vi "Run Tests.vi"(8 "error in (no error)":errorcluster, 10 "Test Cases":refnum<class "Test Case.lvclass">[](array[class]), 11 "LVUnit Test Executor in":refnum<class "LVUnit Test Executor.lvclass">) -> (0 "error out":errorcluster, 2 "Test Results":refnum<class "Test Result.lvclass">[](array[class]), 3 "LVUnit Test Executor out":refnum<class "LVUnit Test Executor.lvclass">)   [LabVIEW 2017, in "LVUnit Test Executor.lvclass"]
doc: "Runs the specified tests."
uses:
  LVUnit Test Executor.lvclass
  Test Case/Test Case.lvclass
  Test Result/Test Result.lvclass
  Test Outcome.ctl
  Test Result/Test Result.lvclass/Test Result.ctl
  Test Result/Set Outcome.vi
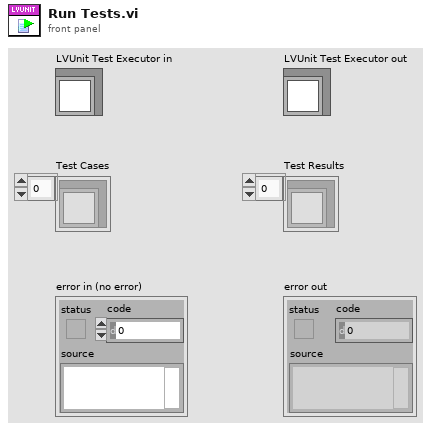
[diagram p1: front panel]
types:
  T1 = typedef "Test Outcome.ctl" = enum16{"None", "Passed", "Failed"}
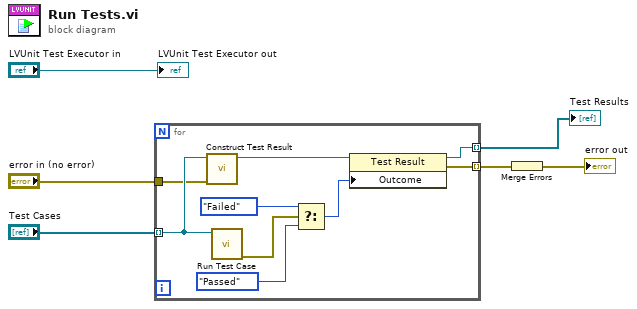
[diagram p0: block diagram]
diagram:
  n1 = for {
    tunnel: "Test Cases" -> [w15] mode=indexing
    tunnel: [w11] -> w4 mode=indexing
    tunnel: "error in (no error)" -> [w14]
    tunnel: [w13] -> w3 mode=indexing
    n2 = call "Construct Test Result.vi"("error in (no error)"=w14, "Test Case"=w15) -> ("Test Result"=w12:refnum<class "Test Result.lvclass">)  [unwired: 8 in, 1 out]
    n3 = call "Run Test Case.vi"("Test Case"=w15) -> ("error out"=w10:errorcluster)  [unwired: 10 in]
    n4 = Select(t=Test_Outcome."Failed" ("Outcome"), s=w10, f=Test_Outcome."Passed" ("Outcome")) -> (s? t:f=w7:T1)
    n5 = property class="Test Result"(reference=w12, "Outcome"=w7) -> (reference out=w11:refnum<class "Test Result.lvclass">, error out=w13:errorcluster)  [unwired: 1 in]
  }
  "Test Results" <- w4
  n6 = Merge Errors(w3) -> (→"error out":errorcluster)
  "LVUnit Test Executor out" <- "LVUnit Test Executor in"
